vi "Initialize.vi"(8 "error in (no error)":errorcluster, 10 "ID Query (True)":bool=TRUE, 11 "VISA resource name":refnum<visa-resource-name>) -> (0 "error out":errorcluster, 3 "VISA resource name out":refnum<visa-resource-name>)   [LabVIEW 2015, in "Micron Optics sm130.lvlib"]
doc: "Establishes communication with the instrument and optionally performs an instrument identification query and/or an instrument reset. It also places the instrument in a default state needed for other instrument driver operations. Therefore, call this VI before calling other instrument driver VIs for this instrument. Generally, you need to call the Initialize VI only once at the beginning of an application."
uses:
  Micron Optics sm130.lvlib
panel:
  # "(c) 2009 - 2012 National Instruments.  ALL RIGHTS RESERVED."
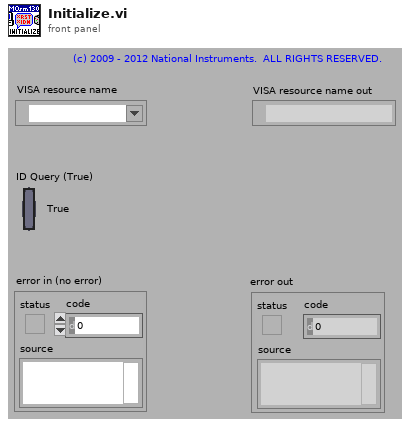
[diagram p1: front panel]
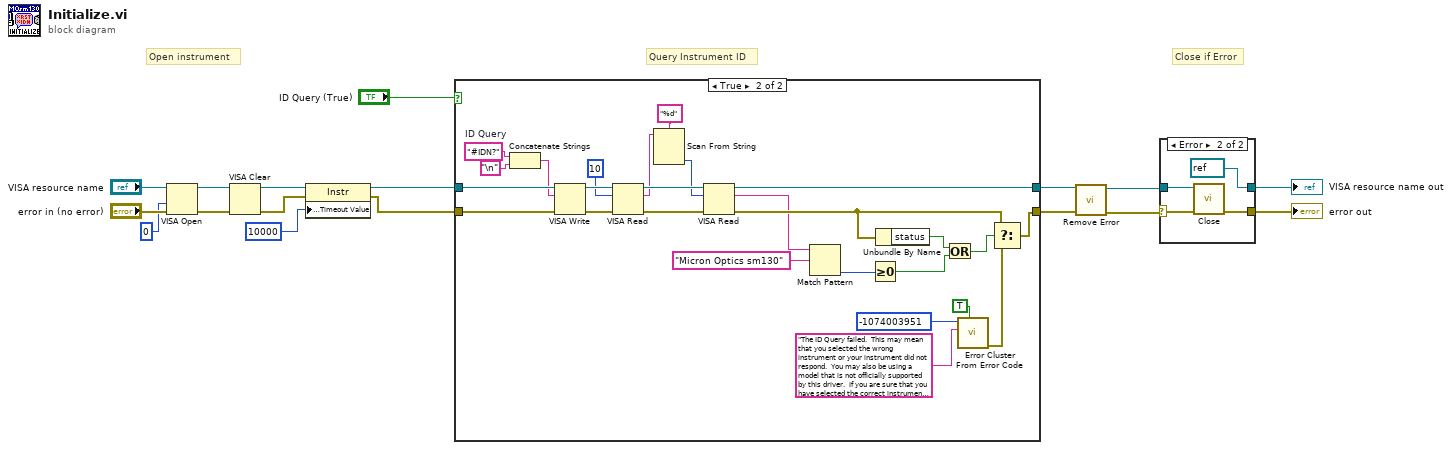
[diagram p0: block diagram]
diagram:
  # "Close if Error"
  # "Query Instrument ID"
  # "Open instrument"
  n1 = VISA Open(access mode=u32 0, error in (no error)="error in (no error)", VISA resource name="VISA resource name") -> (VISA resource name=w12:refnum<visa-resource-name>, error out=w11:errorcluster)  [unwired: 2 in]
  n2 = VISA Clear(VISA resource name=w12, error in (no error)=w11) -> (VISA resource name out=w10:refnum<visa-resource-name>, error out=w9:errorcluster)
  n3 = property class="Instr"(reference=w10, error in=w9, "General Settings:Timeout Value"=u32 10000) -> (reference out=w6:refnum<visa-resource-name>, error out=w5:errorcluster)
  n4 = case shown="True" "ID Query (True)" {
    tunnel: [w18 w45] -> w3
    tunnel: [w19 w28] -> w4
    tunnel: w6 -> [w19 w43]
    tunnel: w5 -> [w18 w44]
    frame False {
    }
    frame True {
      w22 = "#IDN?"  # ID Query
      n5 = Concatenate Strings(w22, "\n") -> (w20:string)
      n6 = VISA Write(VISA resource name=w43, write buffer=w20, error in (no error)=w44) -> (VISA resource name out=w42:refnum<visa-resource-name>, error out=w41:errorcluster)  [unwired: 1 out]
      n7 = VISA Read(VISA resource name=w42, byte count=u32 10, error in (no error)=w41) -> (VISA resource name out=w30:refnum<visa-resource-name>, read buffer=w26:string, error out=w29:errorcluster)  [unwired: 1 out]
      n8 = Scan From String(format string="%d", input string=w26) -> (output 1=w25:i32)  [unwired: 3 in, 3 out]
      n9 = VISA Read(VISA resource name=w30, byte count=w25, error in (no error)=w29) -> (VISA resource name out=w28:refnum<visa-resource-name>, read buffer=w23:string, error out=w27:errorcluster)  [unwired: 1 out]
      n10 = Match Pattern(string=w23, regular expression="Micron Optics sm130") -> (offset past match=w34:i32)  [unwired: 1 in, 3 out]
      n11 = Greater Or Equal To 0?(x=w34) -> (x >= 0?=w32:bool)
      n12 = Unbundle By Name(w27) -> ("status"=w33:bool)
      n13 = Or(x=w33, y=w32) -> (x .or. y?=w31:bool)
      n14 = call <vilib>:"Error Cluster From Error Code.vi"("show call chain? (False)"=TRUE, "error message (\"\")"="The ID Query failed.  This may mean that you selected the wrong instrument or your instrument did not respond.  You may also be using a model that is not officially supported by this driver.  If you are sure that you have selected the correct instrument and it is responding, try disabling the ID Query." ("Source (VI Name)"), "error code (0)"=-1074003951 ("Code")) -> ("error out"=w38:errorcluster)  [unwired: 6 in]
      n15 = Select(t=w27, s=w31, f=w38) -> (s? t:f=w45:errorcluster)
    }
  }
  n16 = call "Remove Error.vi"("error in (no error)"=w3, "VISA resource name"=w4) -> ("error out"=w1:errorcluster, "VISA resource name out"=w2:refnum<visa-resource-name>)  [unwired: 8 in]
  n17 = case shown="Error" w1 {
    selector: w1 -> [w46 w49]
    tunnel: w2 -> [w47 w50]
    tunnel: [w47 refnum<visa-resource-name> refnum ("VISA resource name out")] -> w8
    tunnel: [w46 w51] -> w7
    frame No Error {
    }
    frame Error {
      n18 = call "Close.vi"("error in (no error)"=w49, "VISA resource name"=w50) -> ("error out"=w51:errorcluster)  [unwired: 9 in]
    }
  }
  "VISA resource name out" <- w8
  "error out" <- w7
